vi "LabVIEW Data to Python String (I8 Array).vi"(8 "error in (no error)":errorcluster, 10 "LabVIEW Data":i8[](array[numeric])) -> (0 "error out":errorcluster, 2 "Python String":string)   [LabVIEW 2020, in "jki_python_data_tools.lvlib"]
doc: "Writes a value associated with key in a specified section of the configuration data identified by refnum. If \"key\" input is not specified, the name of the variant object is used as the key.\n\nFor example a Boolean named \"Enable\" with a value of TRUE would correspond to the key-value pair:\n\nEnable=TRUE"
uses:
  jki_python_data_tools.lvlib
panel:
  # "Copyright © 2003-2009 JKI. All rights reserved.\n\nAuthor: Jim Kring [jim.kring@jameskring.com]\n\nThis library is provided \"AS IS\" ,WITHOUT WARRANTIES OR \nCONDITIONS OF ANY KIND, either express or implied.\n\nJames Kring, Inc. -- http://www.jameskring.com"
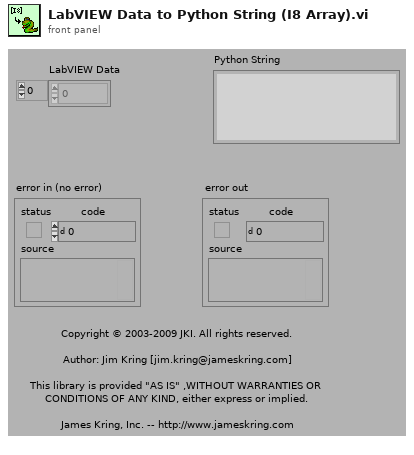
[diagram p1: front panel]
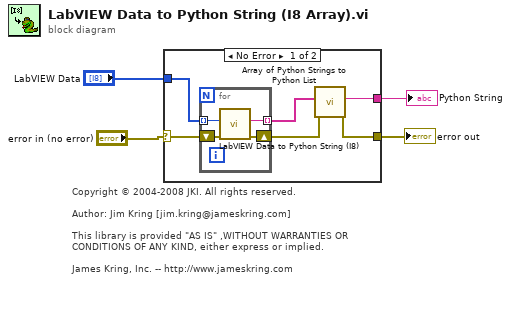
[diagram p0: block diagram]
diagram:
  # "Copyright © 2004-2008 JKI. All rights reserved.\n\nAuthor: Jim Kring [jim.kring@jameskring.com]\n\nThis library is provided \"AS IS\" ,WITHOUT WARRANTIES OR \nCONDITIONS OF ANY KIND, either express or implied.\n\nJames Kring, Inc. -- http://www.jameskring.com"
  n1 = case shown="No Error" "error in (no error)" {
    selector: "error in (no error)" -> [w9 w15]
    tunnel: "LabVIEW Data" -> [w10 _]
    tunnel: [w7 _] -> w2
    tunnel: [w5 w15] -> w3
    frame No Error {
      n2 = for {
        tunnel: w10 -> [w14] mode=indexing
        shift-right: [w12] -> w6
        shift-left: w9 -> [w13]
        tunnel: [w11] -> w8 mode=indexing
        n3 = call "LabVIEW Data to Python String (I8).vi"("error in (no error)"=w13, "LabVIEW Data"=w14) -> ("error out"=w12:errorcluster, "Python String"=w11:string)  [unwired: 8 in]
      }
      n4 = call "Array of Python Strings to Python List.vi"("error in (no error)"=w6, "Array of Python Strings"=w8) -> ("error out"=w5:errorcluster, "Python List"=w7:string)  [unwired: 8 in]
    }
    frame Error {
    }
  }
  "error out" <- w3
  "Python String" <- w2
